vi "Manual Override.vi"(7 "Velocity":dbl, 8 "Override":enum32{"None", "Velocity", "Position", "STOP"}(ring), 9 "Counts":i32, 10 "Position GO":bool, 11 "Auto CMD":T1) -> (2 "Position GO Out":bool, 3 "OverRide Command Out":T1, 5 "Velocity Out":dbl)   [LabVIEW 2020, in "Wrist_ACT.lvlib"]
uses:
  Wrist_ACT.lvlib
  Cluster_CMD_ACT_Data.ctl
  Shared Code/TypeDefs/ENUM_Wrist_CMD_Mode Select.ctl
  Extention/Cluster_CMD_ACT_Data.ctl
  Shared Code/TypeDefs/ENUM_Extend_CMD_Mode Select.ctl
  Extention/Extend_ACT.lvlib
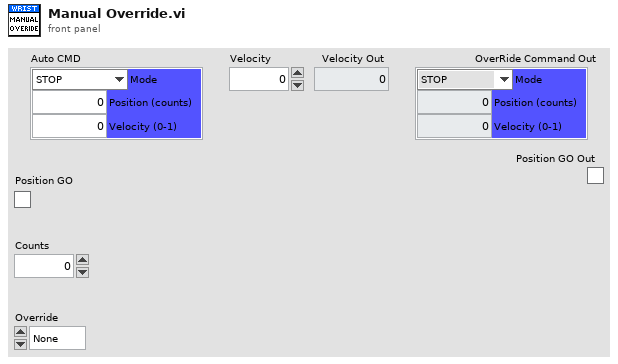
[diagram p1: front panel]
types:
  T1 = typedef "Wrist_ACT.lvlib/Cluster_CMD_ACT_Data.ctl" = cluster{"Mode":T2, "Position (counts)":i32, "Velocity (0-1)":dbl}
  T2 = typedef "ENUM_Wrist_CMD_Mode Select.ctl" = enum16{"STOP", "Position", "Velocity"}
  T3 = typedef "Extend_ACT.lvlib/Cluster_CMD_ACT_Data.ctl" = cluster{"Mode":T4, "Position (counts)":i32, "Velocity (0-1)":dbl}
  T4 = typedef "ENUM_Extend_CMD_Mode Select.ctl" = enum16{"STOP", "Position", "Velocity", "Force Home"}
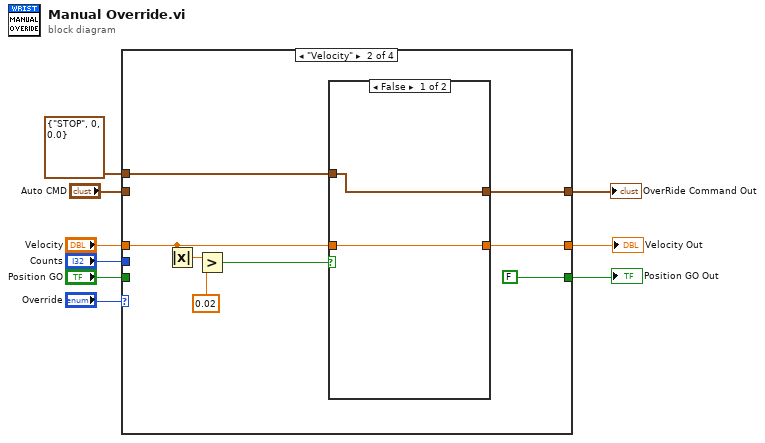
[diagram p0: block diagram]
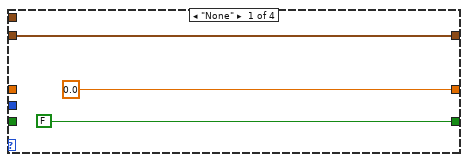
[diagram p2: hidden frame]
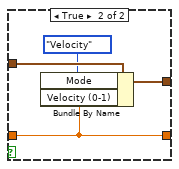
[diagram p3: hidden frame]
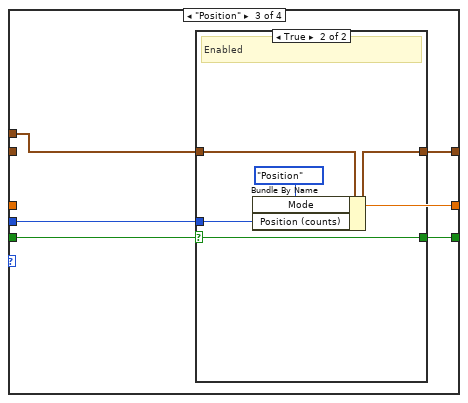
[diagram p4: hidden frame]
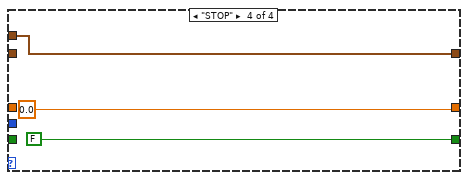
[diagram p6: hidden frame]
diagram:
  n1 = case shown="\"Velocity\"" "Override" {
    tunnel: [w10 w17 w31 w42] -> w9
    tunnel: T3 {"Mode"=enum."STOP", "Position (counts)"=0, "Velocity (0-1)"=0.0} ("CMD_ExtendTemplate_Data 3") -> [_ w18 w32 w42]
    tunnel: "Counts" -> [_ _ w30 _]
    tunnel: [0.0 ("Velocity") w14 0.0 ("Velocity") 0.0 ("Velocity")] -> w4
    tunnel: "Position GO" -> [_ _ w28 _]
    tunnel: [FALSE FALSE w27 FALSE] -> w6
    tunnel: "Velocity" -> [_ w16 _ _]
    tunnel: "Auto CMD" -> [w10 _ _ _]
    frame "None" {
    }
    frame "Velocity" {
      n2 = Absolute Value(x=w16) -> (abs(x)=w13:dbl)
      n3 = Greater?(x=w13, y=0.02) -> (0:w19:bool)
      n4 = case shown="False" w19 {
        tunnel: w18 -> [w22 w26]
        tunnel: [w22 w25] -> w17
        tunnel: w16 -> [w21 w24]
        tunnel: [w21 w24] -> w14
        frame False {
        }
        frame True {
          n5 = Bundle By Name(cluster=w26, "Mode"=ENUM_Extend_CMD_Mode_Select."Velocity", "Velocity (0-1)"=w24) -> (w25:T3)
        }
      }
    }
    frame "Position" {
      n6 = case shown="True" w28 {
        selector: w28 -> [w33 w36]
        tunnel: w32 -> [w34 w39]
        tunnel: [w34 w38] -> w31
        tunnel: w30 -> [_ w37]
        tunnel: [w33 w36] -> w27
        frame False {
          # "Disabled"
        }
        frame True {
          # "Enabled"
          n7 = Bundle By Name(cluster=w39, "Mode"=ENUM_Extend_CMD_Mode_Select."Position", "Position (counts)"=w37) -> (w38:T3)
        }
      }
    }
    frame "STOP" {
    }
  }
  "OverRide Command Out" <- w9
  "Position GO Out" <- w6
  "Velocity Out" <- w4
